vi "SendStatus.vi"(8 "error in (no error)":errorcluster, 11 "Instrument in":refnum<class "Instrument.lvclass">) -> (0 "error out":errorcluster, 3 "Instrument out":refnum<class "Instrument.lvclass">)   [LabVIEW 2018, in "Instrument.lvclass"]
uses:
  Instrument.lvclass
  Server/Server.lvclass
  Comm/Stream/Stream.lvclass
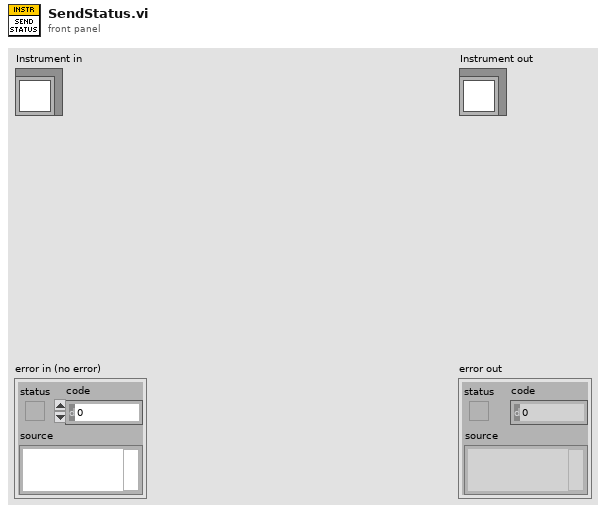
[diagram p1: front panel]
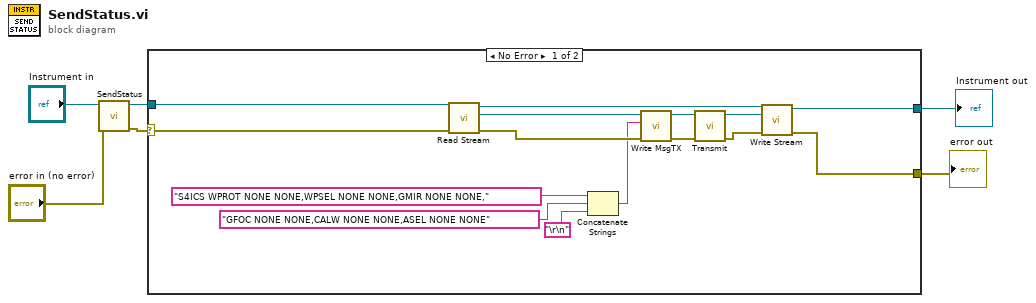
[diagram p0: block diagram]
diagram:
  n1 = call-parent "SendStatus.vi"("error in (no error)"="error in (no error)", "Server in"="Instrument in") -> ("error out"=w3:errorcluster, "Server out"=w4:refnum<class "Instrument.lvclass">)  [unwired: 8 in]
  n2 = case shown="No Error" w3 {
    selector: w3 -> [w14 w22]
    tunnel: w4 -> [w17 w23]
    tunnel: [w15 w23] -> w2
    tunnel: [w7 w22] -> w1
    frame No Error {
      n3 = call-dynamic "Read Stream.vi"("error in (no error)"=w14, "Server in"=w17) -> ("error out"=w13:errorcluster, "Stream.lvclass"=w12:refnum<class "Stream.lvclass">, "Server out"=w16:refnum<class "Instrument.lvclass">)  [unwired: 7 in]
      n4 = Concatenate Strings("S4ICS WPROT NONE NONE,WPSEL NONE NONE,GMIR NONE NONE," ("MsgTX"), "GFOC NONE NONE,CALW NONE NONE,ASEL NONE NONE" ("MsgTX"), "\r\n" ("string")) -> (w8:string)
      n5 = call-dynamic "Write MsgTX.vi"("error in (no error)"=w13, "MsgTX"=w8, "Comm in"=w12) -> ("error out"=w20:errorcluster, "Comm out"=w21:refnum<class "Stream.lvclass">)  [unwired: 7 in]
      n6 = call-dynamic "Transmit.vi"("error in (no error)"=w20, "Stream in"=w21) -> ("error out"=w18:errorcluster, "Stream out"=w19:refnum<class "Stream.lvclass">)  [unwired: 8 in]
      n7 = call-dynamic "Write Stream.vi"("error in (no error)"=w18, "Stream.lvclass"=w19, "Server in"=w16) -> ("error out"=w7:errorcluster, "Server out"=w15:refnum<class "Instrument.lvclass">)  [unwired: 7 in]
    }
    frame Error {
    }
  }
  "error out" <- w1
  "Instrument out" <- w2
